vi "Initialize.vi"(2 "error in (no error)":errorcluster, 4 "Data In":T1 {"Shaft"."dmin" format="%#_7g"; "Shaft"."dmax" format="%#_7g"; "Shaft"."Fundamental Dev" format="%#_7g"; "Shaft"."Tolerance Grade (IT) Shaft" format="%#_7g"; "Hole"."Dmin" format="%#_7g"; "Hole"."Tolerance Grade (IT)" format="%#_7g"}) -> (0 "error out":errorcluster, 1 "Data Out":T1 {"Shaft"."dmin" format="%#_7g"; "Shaft"."dmax" format="%#_7g"; "Shaft"."Fundamental Dev" format="%#_7g"; "Shaft"."Tolerance Grade (IT) Shaft" format="%#_7g"; "Hole"."Dmin" format="%#_7g"; "Hole"."Tolerance Grade (IT)" format="%#_7g"})   [LabVIEW 2023]
uses:
  TypeDef/Data_Cluster.ctl
  TypeDef/Units.ctl
  TypeDef/Method_Info.ctl
  TypeDef/Hole_Data.ctl
  TypeDef/Shaft_Data.ctl
  <vilib>/Utility/config.llb/Read Key (Path).vi
  <vilib>/Utility/config.llb/NI_LVConfig.lvlib
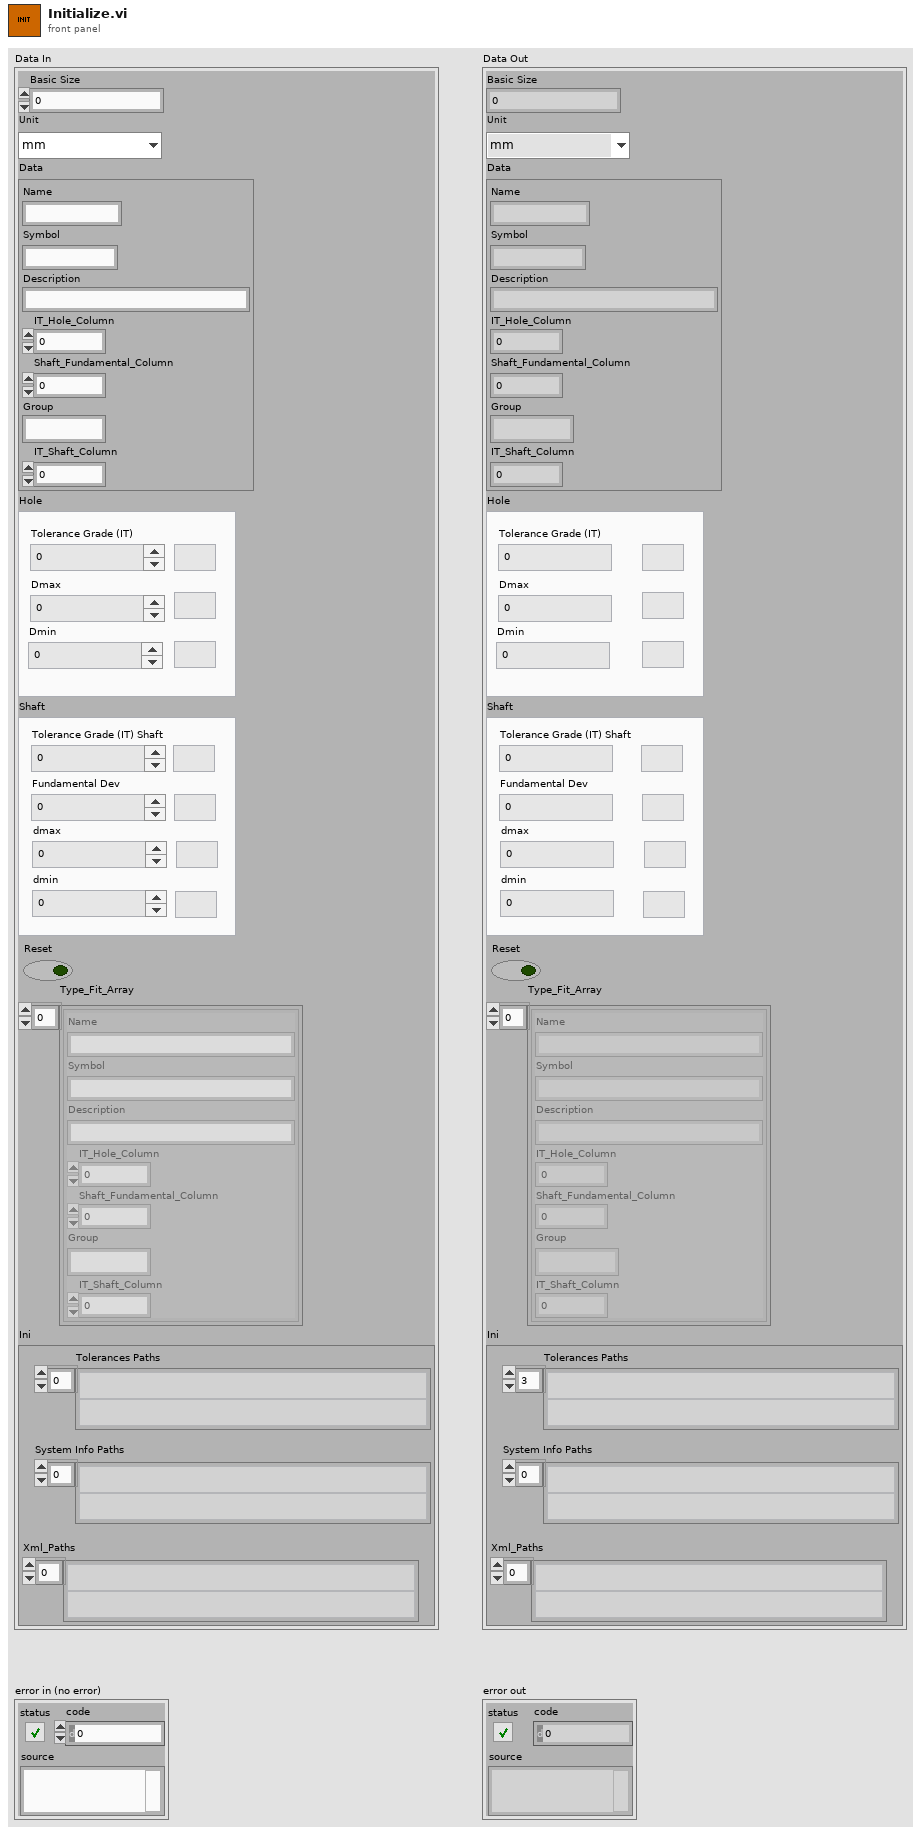
[diagram p1: front panel]
types:
  T1 = typedef "Data_Cluster.ctl" = cluster{"Basic Size ":dbl, "Unit":T2, "Data":T3, "Hole":T4, "Shaft":T5, "Reset":bool, "Type_Fit_Array":T3[], "Ini":cluster{"Tolerances Paths":path[], "System Info Paths":path[], "Xml_Paths":path[]}}
  T2 = typedef "Units.ctl" = enum16{"mm", "in"}
  T3 = typedef "Method_Info.ctl" = cluster{"Name":string, "Symbol":string, "Description":string, "IT_Hole_Column":i32, "Shaft_Fundamental_Column":i32, "Group":string, "IT_Shaft_Column":i32}
  T4 = typedef "Hole_Data.ctl" = cluster{"Tolerance Grade (IT)":dbl, "Dmax":dbl, "Units Hole":cluster{"units_it":string, "units_Dmax\nUnits_Dmax":string, "Units_Dmin":string}, "Dmin":dbl}
  T5 = typedef "Shaft_Data.ctl" = cluster{"Tolerance Grade (IT) Shaft":dbl, "Units Shaft":cluster{"Units_FundamentalDev":string, "Units_dmax":string, "Units_dmin":string, "Units_IT_Shaft":string}, "Fundamental Dev":dbl, "dmax":dbl, "dmin":dbl}
  T6 = typedef "NI_LVConfig.lvlib/Config Data RefNum.ctl" = refnum<k1>
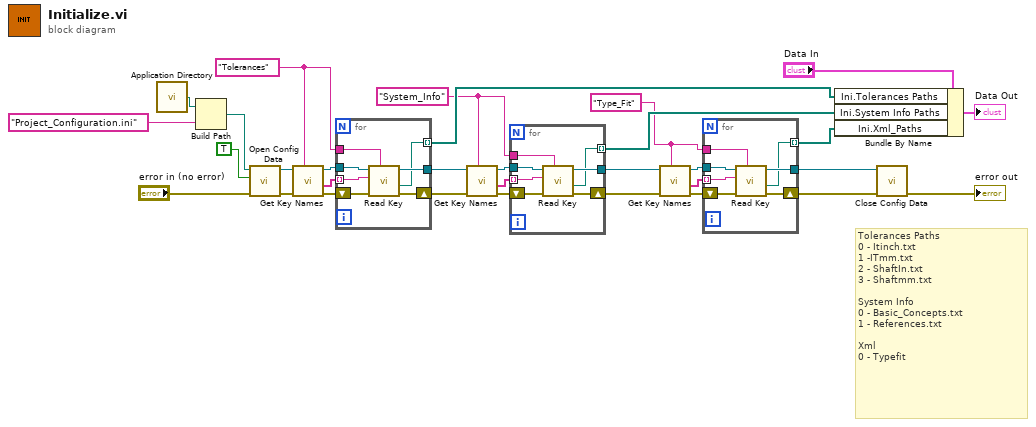
[diagram p0: block diagram]
diagram:
  w4 = "Type_Fit"
  w10 = "System_Info" ("section")
  w23 = "Tolerances"
  # "Tolerances Paths\n0 - Itinch.txt\n1 -ITmm.txt\n2 - ShaftIn.txt\n3 - Shaftmm.txt\n\nSystem Info \n0 - Basic_Concepts.txt\n1 - References.txt\n\nXml\n0 - Typefit"
  n1 = call <vilib>:"Application Directory.vi"() -> ("Application Directory"=w30:path)
  n2 = Build Path(base path=w30, name or relative path="Project_Configuration.ini") -> (appended path=w18:path)
  n3 = call <vilib>:"Open Config Data.vi"("error in (no error)"="error in (no error)", "create file if necessary (T)"=TRUE, "configuration file path"=w18) -> ("error out"=w28:errorcluster, "refnum"=w27:T6)  [unwired: 6 in, 1 out]
  n4 = call <vilib>:"Get Key Names.vi"("section"=w23, "error in (no error)"=w28, "refnum"=w27) -> ("error out"=w26:errorcluster, "key names"=w24:string[], "refnum out"=w25:T6)  [unwired: 5 in, 1 out]
  n5 = for {
    shift-right: [w37] -> w15
    shift-left: w26 -> [w38]
    tunnel: w25 -> [w36]
    tunnel: w24 -> [w35] mode=indexing
    tunnel: w23 -> [w34]
    tunnel: [w33] -> w13
    tunnel: [w32] -> w19 mode=indexing
    n6 = call-poly <vilib>:"Read Key.vi"("section"=w34, "error in (no error)"=w38, "key"=w35, "refnum"=w36) -> ("error out"=w37:errorcluster, "value"=w32:path, "refnum out"=w33:T6)  [unwired: 4 in, 1 out]
  }
  n7 = call <vilib>:"Get Key Names.vi"("section"=w10, "error in (no error)"=w15, "refnum"=w13) -> ("error out"=w14:errorcluster, "key names"=w11:string[], "refnum out"=w12:T6)  [unwired: 5 in, 1 out]
  n8 = for {
    shift-right: [w44] -> w9
    shift-left: w14 -> [w45]
    tunnel: w12 -> [w43]
    tunnel: [w42] -> w8
    tunnel: [w41] -> w16 mode=indexing
    tunnel: w11 -> [w40] mode=indexing
    tunnel: w10 -> [w39]
    n9 = call-poly <vilib>:"Read Key.vi"("section"=w39, "error in (no error)"=w45, "key"=w40, "refnum"=w43) -> ("error out"=w44:errorcluster, "value"=w41:path, "refnum out"=w42:T6)  [unwired: 4 in, 1 out]
  }
  n10 = call <vilib>:"Get Key Names.vi"("section"=w4, "error in (no error)"=w9, "refnum"=w8) -> ("error out"=w7:errorcluster, "key names"=w5:string[], "refnum out"=w1:T6)  [unwired: 5 in, 1 out]
  n11 = for {
    shift-right: [w51] -> w6
    shift-left: w7 -> [w52]
    tunnel: [w50] -> w2
    tunnel: [w49] -> w3 mode=indexing
    tunnel: w5 -> [w48] mode=indexing
    tunnel: w4 -> [w47]
    tunnel: w1 -> [w46]
    n12 = call-poly <vilib>:"Read Key.vi"("section"=w47, "error in (no error)"=w52, "key"=w48, "refnum"=w46) -> ("error out"=w51:errorcluster, "value"=w49:path, "refnum out"=w50:T6)  [unwired: 4 in, 1 out]
  }
  n13 = Bundle By Name(cluster="Data In", "Ini.Tolerances Paths"=w19, "Ini.System Info Paths"=w16, "Ini.Xml_Paths"=w3) -> (→"Data Out":T1)
  n14 = call <vilib>:"Close Config Data.vi"("error in (no error)"=w6, "refnum"=w2) -> ("error out"=→"error out":errorcluster)  [unwired: 8 in, 1 out]
